vi "CSDB_Transfer.get instance data from DB.vi"(4 "error in (no error)":errorcluster, 6 "Instance":string, 7 "Data source":string) -> (0 "error out":errorcluster, 2 "from DB instance":string[](array[string]), 3 "from DB data":string[][](array[string]))   [LabVIEW 2014, in "CSDB_Transfer.lvlib"]
doc: "Opens a connection to the database and reads the data of one instance."
uses:
  CSDB_Transfer.lvlib
  <vilib>/addons/database/Connection.llb/DB Tools Open Connec (String).vi
  <vilib>/addons/database/NI_Database_API.lvlib
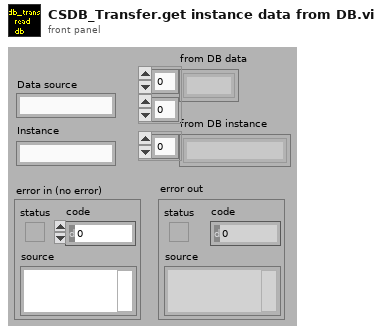
[diagram p1: front panel]
types:
  T1 = typedef "NI_Database_API.lvlib/Conn ObjectReference.ctl" = refnum<k1>
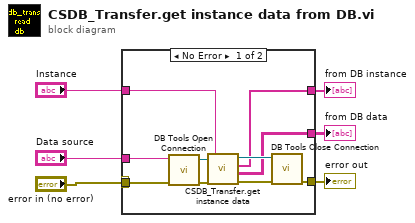
[diagram p0: block diagram]
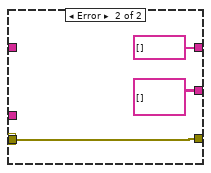
[diagram p2: hidden frame]
diagram:
  n1 = case shown="No Error" "error in (no error)" {
    selector: "error in (no error)" -> [_ w19]
    tunnel: [w16 w19] -> w6
    tunnel: [w11 string[] [] ("InstanceName      Classname")] -> w5
    tunnel: [w10 string[][] [] ("InstanceName      AttributeName      Value")] -> w4
    tunnel: "Data source" -> [w9 _]
    tunnel: "Instance" -> [w8 _]
    tunnel: "error in (no error)" -> [w7 _]
    frame No Error {
      n2 = call-poly <vilib>:"DB Tools Open Connection.vi"("error in (no error)"=w7, "connection information"=w9) -> ("error out"=w14:errorcluster, "connection reference"=w15:T1)  [unwired: 6 in]
      n3 = call "CSDB_Transfer.get instance data.vi"("connection reference"=w15, "InstanceName"=w8, "error in (no error)"=w14) -> ("connection reference out"=w13:T1, "InstanceName      Classname"=w11:string[], "InstanceName      AttributeName      Value"=w10:string[][], "error out"=w12:errorcluster)
      n4 = call <vilib>:"DB Tools Close Connection.vi"("error in (no error)"=w12, "connection reference"=w13) -> ("error out"=w16:errorcluster)  [unwired: 5 in]
    }
    frame Error {
    }
  }
  "error out" <- w6
  "from DB instance" <- w5
  "from DB data" <- w4
